vi "Read_GEA3.vi"(0 "session in":refnum<k35>, 7 "dst":i64 format="%x", 9 "ERD":i64 format="%x", 11 "error in (no error)":errorcluster) -> (4 "session out":refnum<k35>, 8 "Read ERD":T1 {"ERD Number" format="%x"}, 15 "error out":errorcluster)   [LabVIEW 2021]
uses:
  Controles/Read_ERD.ctl
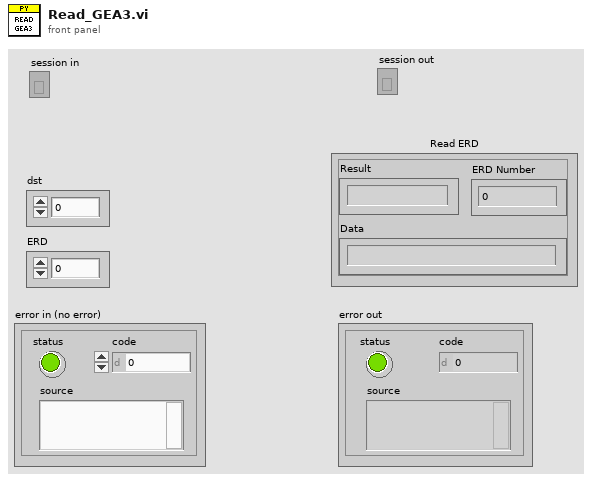
[diagram p1: front panel]
types:
  T1 = typedef "Read_ERD.ctl" = cluster{"Result":string, "ERD Number":i64, "Data":string}
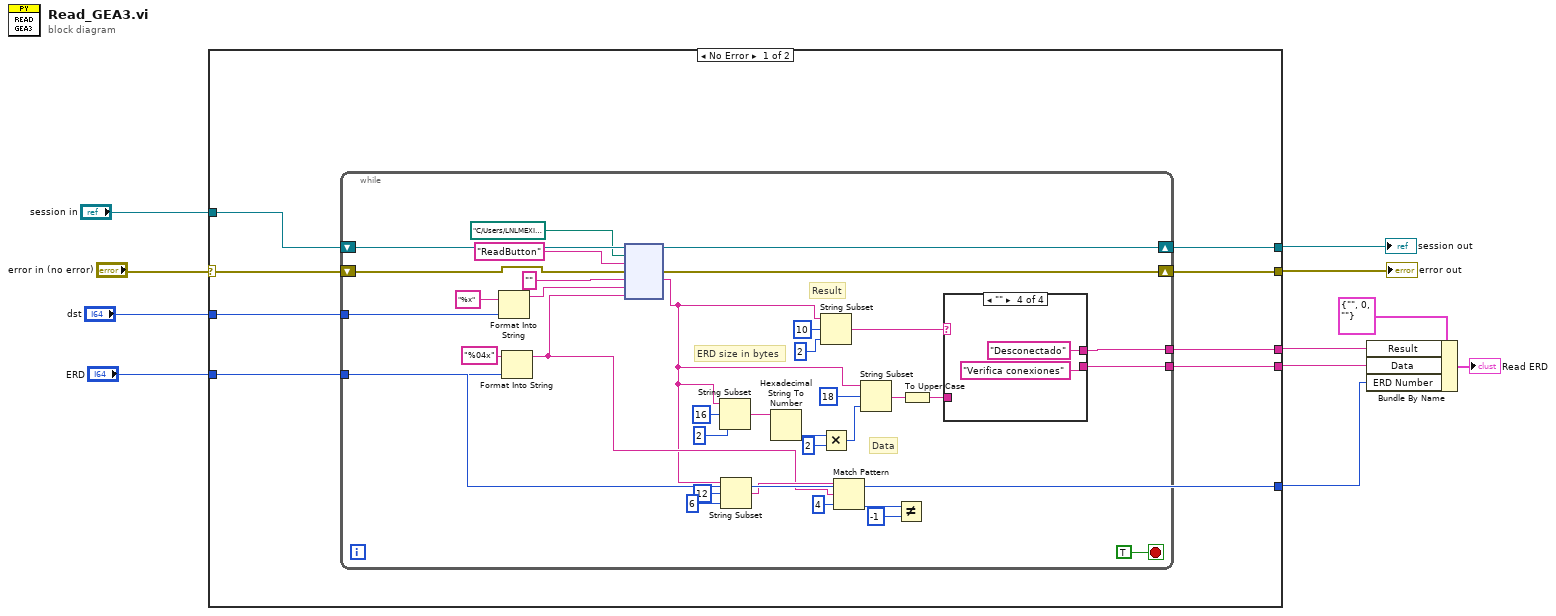
[diagram p0: block diagram]
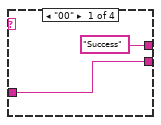
[diagram p2: hidden frame]
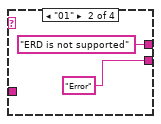
[diagram p3: hidden frame]
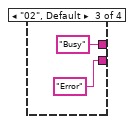
[diagram p4: hidden frame]
diagram:
  n1 = case shown="No Error" "error in (no error)" {
    selector: "error in (no error)" -> [w14 w64]
    tunnel: "dst" -> [w19 _]
    tunnel: "ERD" -> [w12 _]
    tunnel: "session in" -> [w18 w63]
    tunnel: [w17 w63] -> w8
    tunnel: [w16 w64] -> w7
    tunnel: [w15 _] -> w6
    tunnel: [w13 _] -> w2
    tunnel: [w12 _] -> w1
    frame No Error {
      n2 = while {
        tunnel: w19 -> [w54]
        tunnel: [w50] -> w15
        tunnel: [w31] -> w13
        tunnel: w12 -> [w30]
        shift-right: [w52] -> w17
        shift-left: w18 -> [w53]
        shift-right: [w51] -> w16
        shift-left: w14 -> [w34]
        stop <- TRUE stop-if-true
        # "Data"
        # "Result"
        # "ERD size in bytes"
        n3 = Format Into String(format string="%x", w54) -> (resulting string=w46:string)  [unwired: 2 in, 1 out]
        n4 = Format Into String(format string="%04x", w30) -> (resulting string=w24:string)  [unwired: 2 in, 1 out]
        n5 = node(w53, path "C:/Users/LNLMEXID/Desktop/GEA3 Python/Main.py" ("module path"), "ReadButton" ("function name"), w34, "" ("data_hex"), w46, w24) -> (w52:refnum<k35>, w51:errorcluster, w23:string)  [unwired: 2 in, 2 out]
        n6 = String Subset(string=w23, offset (0)=16, length (rest)=2 ("length (rest)")) -> (substring=w39:string)
        n7 = String Subset(string=w23, offset (0)=12, length (rest)=6 ("length (rest)")) -> (substring=w25:string)
        n8 = Hexadecimal String To Number(string=w39) -> (number=w36:u32)  [unwired: 2 in, 1 out]
        n9 = String Subset(string=w23, offset (0)=10, length (rest)=2 ("length (rest)")) -> (substring=w42:string)
        n10 = Multiply(x=w36, y=u32 2) -> (x*y=w35:u32)
        n11 = Match Pattern(string=w25, regular expression=w24, offset (0)=4) -> (offset past match=w28:i32)  [unwired: 3 out]
        n12 = String Subset(string=w23, offset (0)=18, length (rest)=w35) -> (substring=w33:string)
        n13 = Not Equal?(x=w28, y=-1) -> ()  [unwired: 1 out]
        n14 = To Upper Case(1:w33) -> (0:w32:string)
        n15 = case shown="\"\"" w42 {
          tunnel: ["Success" "ERD is not supported" "Busy" "Desconectado"] -> w50
          tunnel: w32 -> [w55 _ _ _]
          tunnel: [w55 "Error" "Error" "Verifica conexiones"] -> w31
          frame "00" {
          }
          frame "01" {
          }
          frame "02", Default {
          }
          frame "" {
          }
        }
      }
    }
    frame Error {
    }
  }
  "session out" <- w8
  "error out" <- w7
  n16 = Bundle By Name(cluster=T1 {"Result"="", "ERD Number"=0, "Data"=""} ("Read ERD"), "Result"=w6, "Data"=w2, "ERD Number"=w1) -> (→"Read ERD":T1)
